vi "Z_info_Save.vi"(7 "Zplane in":i32, 8 "error in (no error)":errorcluster, 11 "AOL_Globals":T1={"Imaging Protocol"=enum."AOL Z-Stack", "Number of POI"=0, "Number of Miniscans"=0, "Number of Trials"=0, "Number of Cycles "=0, "# Averaged Frames"=0, "Laser power (%)"=0, "Pockels"=0.0, "Acquisition Length (sec)"=0.0, "Fill time (us)"=0.0, "POI Dwell time (us)"=0.0, "Miniscan Dwell time per pixel (us)"=0.0, "PMT 1"=0.0, "PMT 2"=0.0, "Back Apperture"=200.0, "Frame Size"=0, "Center Frequency"=0.0, "Field of View"=0.0, "DwellTime (us)"=0.0, "Wavelength (nm)"=0.0, "Zoom"=0.0, "AOL Z"=0.0, "AOL Mode"=enum."Raster", "GridXY"=0.0, "GridZ"=0.0, "TriggerPeriod (sec)"=0.0, "Number of Pixels in Miniscan"=0, "Experiment folder path"=path "", "X centre"=0.0, "Y centre"=0.0, "Angle (degrees)"=0.0, "Plane Mode"=0, "Threshold"=[], "Regenerate Chirps"=FALSE, "Rectangle ROI length (pixels)"=0, "Rectangle ROI height (pixels)"=0, "AOD fill"=0, "Samples Wait after Trigger"=0, "StartUp Delay"=0, "Slip Cycle"=163840, "Add Cycle"=FALSE} {"Plane Mode" items=["XY Plane"]; "Frame Size" items=["100X100"=100, "128X128"=128, "200X200"=200, "256X256"=256, "512X512"=512, "1024x1024"=1024, "2048x2048"=2048]; "Back Apperture" format="%#.6g"; "Pockels" format="%#.6g"; "PMT 2" format="%#.6g"; "PMT 1" format="%#.6g"; "Angle (degrees)" format="%#.6g"; "POI Dwell time (us)" format="%#.6g"}) -> (0 "error out":errorcluster)   [LabVIEW 2013]
uses:
  Typedefs/Controls/AOL_Globals.ctl
  Typedefs/Imaging Protocols enum.ctl
  Typedefs/Frame Size.ctl
  Typedefs/AOL modes.ctl
  Typedefs/Plane Mode.ctl
  <userlib>/My Palettes.lib/Files & paths/Spreadsheet/Write To Spreadsheet File (DBL)-Mod.vi
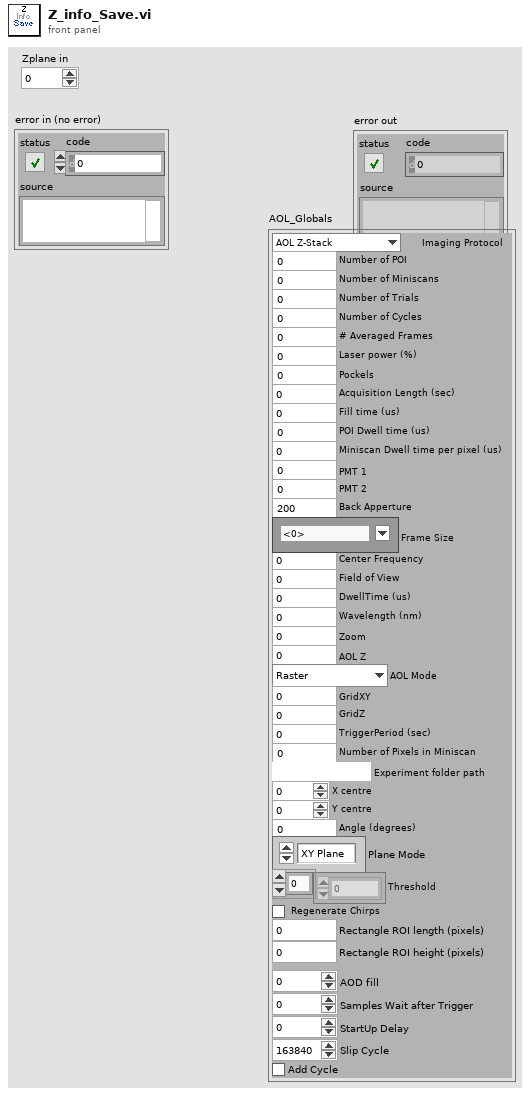
[diagram p1: front panel]
types:
  T1 = typedef "AOL_Globals.ctl" = cluster{"Imaging Protocol":T2, "Number of POI":u16, "Number of Miniscans":u16, "Number of Trials":u16, "Number of Cycles ":u64, "# Averaged Frames":u16, "Laser power (%)":u8, "Pockels":dbl, "Acquisition Length (sec)":dbl, "Fill time (us)":dbl, "POI Dwell time (us)":dbl, "Miniscan Dwell time per pixel (us)":dbl, "PMT 1":dbl, "PMT 2":dbl, "Back Apperture":dbl, "Frame Size":T3, "Center Frequency":dbl, "Field of View":dbl, "DwellTime (us)":dbl, "Wavelength (nm)":dbl, "Zoom":dbl, "AOL Z":dbl, "AOL Mode":T4, "GridXY":dbl, "GridZ":dbl, "TriggerPeriod (sec)":dbl, "Number of Pixels in Miniscan":u16, "Experiment folder path":path, "X centre":dbl, "Y centre":dbl, "Angle (degrees)":dbl, "Plane Mode":T5, "Threshold":u16[], "Regenerate Chirps":bool, "Rectangle ROI length (pixels)":u16, "Rectangle ROI height (pixels)":u16, "AOD fill":u16, "Samples Wait after Trigger":u16, "StartUp Delay":i32, "Slip Cycle":u32, "Add Cycle":bool}
  T2 = typedef "Imaging Protocols enum.ctl" = enum16{"AOL Z-Stack", "Motor Z Stack", "Functional Acquisition", "Single Plane Acquisition", "Volume Acquisition", "Live Imaging", "Live Plane Imaging", "Live Volume Imaging"}
  T3 = typedef "Frame Size.ctl" = u16
  T4 = typedef "AOL modes.ctl" = enum16{"Raster", "Structural", "Pointing", "Mini Scan", "Alignment"}
  T5 = typedef "Plane Mode.ctl" = u16
  T6 = typedef "Fixed strings.ctl" = cluster{"ROI file name":string, "Normalised ROI file name":string, "Zplane Pockels values file name":string, "Functional data folder name":string, "Experiment Header file name":string, "Z-stack images folder name":string, "Groups setup rel. path":string, "Groups text file rel. path":string, "TDMS files folder name (F.img)":string, "TDMS files folder name (V.acq)":string, "TDMS files folder name (Pl.acq)":string, "Cycle rel times sequence file":string, "Dynamically called VIs folder name":string, "Time Series folder base name":string}
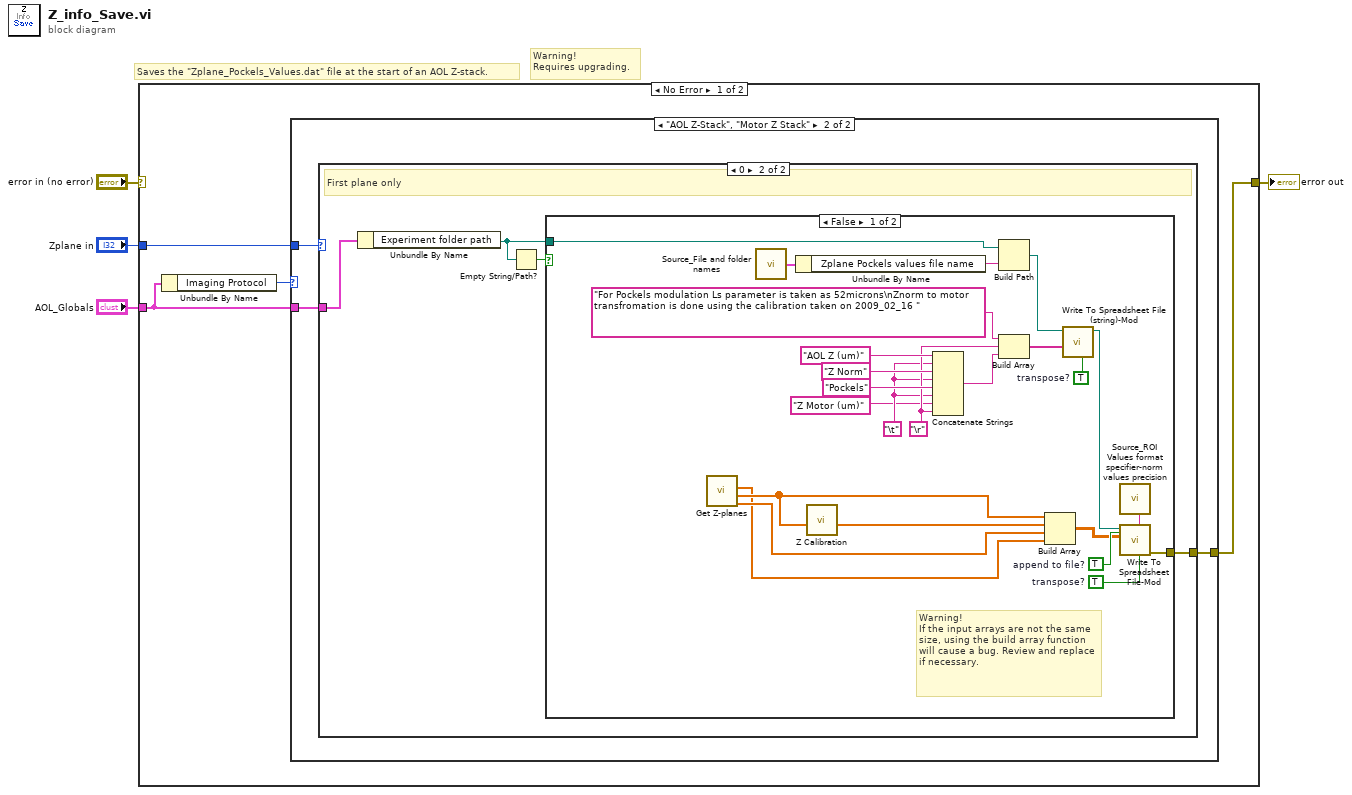
[diagram p0: block diagram]
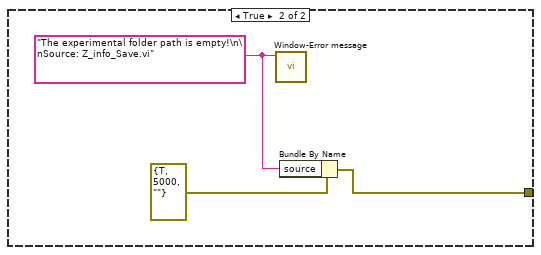
[diagram p4: hidden frame]
diagram:
  # "Warning!\nRequires upgrading."
  # "Saves the \"Zplane_Pockels_Values.dat\" file at the start of an AOL Z-stack."
  n1 = case shown="No Error" "error in (no error)" {
    selector: "error in (no error)" -> [_ w43]
    tunnel: [w5 w43] -> w3
    tunnel: "Zplane in" -> [w7 _]
    tunnel: "AOL_Globals" -> [w6 _]
    frame No Error {
      n2 = Unbundle By Name(w6) -> ("Imaging Protocol"=w8:T2)
      n3 = case shown="\"AOL Z-Stack\", \"Motor Z Stack\"" w8 {
        tunnel: w7 -> [_ w11]
        tunnel: w6 -> [_ w10]
        tunnel: [_ w9] -> w5
        frame Default {
          # "Any protocol other than AOL and Motor Z-stack."
        }
        frame "AOL Z-Stack", "Motor Z Stack" {
          n4 = case shown="0" w11 {
            tunnel: w10 -> [_ w15]
            tunnel: [_ w12] -> w9
            frame Default {
              # "Any plane other than the first one."
            }
            frame 0 {
              # "First plane only"
              n5 = Unbundle By Name(w15) -> ("Experiment folder path"=w14:path)
              n6 = Empty String/Path?(string/path=w14) -> (empty?=w13:bool)
              n7 = case shown="False" w13 {
                tunnel: w14 -> [w37 _]
                tunnel: [w16 w41] -> w12
                frame False {
                  w39 = TRUE  # transpose?
                  w38 = TRUE  # transpose?
                  w33 = TRUE  # append to file?
                  w21 = "\r" ("string")
                  w20 = "\t" ("string")
                  # "Warning!\nIf the input arrays are not the same size, using the build array function will cause a bug. Review and replace if necessary."
                  n8 = call "Get Z-planes.vi"() -> ("Pockels vs. Z (Laser power %)"=w22:dbl[], "Z Planes(um)"=w23:dbl[], "Motor Z Planes(um)"=w17:dbl[])  [unwired: 7 in, 2 out]
                  n9 = call "Source_File and folder names.vi"() -> ("Fixed strings"=w34:T6)  [unwired: 1 in]
                  n10 = Unbundle By Name(w34) -> ("Zplane Pockels values file name"=w35:string)
                  n11 = call "Z Calibration.vi"("Z Planes"=w23) -> ("Norm Z"=w18:dbl[])  [unwired: 7 in, 3 out]
                  n12 = Concatenate Strings("AOL Z (um)" ("string"), w20, "Z Norm" ("string"), w20, "Pockels" ("string"), w20, "Z Motor (um)" ("string"), w21) -> (w27:string)
                  n13 = Build Path(base path=w37, name or relative path=w35) -> (appended path=w32:path)
                  n14 = Build Array("For Pockels modulation Ls parameter is taken as 52microns\nZnorm to motor transfromation is done using the calibration taken on 2009_02_16 " ("element"), w21, w27) -> (w28:string[])
                  n15 = Build Array(w23, w18, w22, w17) -> (w31:dbl[][])
                  n16 = call <userlib>:"Write To Spreadsheet File (string)-Mod.vi"("transpose? (no:F)"=w38, "1D data"=w28, "file path (dialog if empty)"=w32) -> ("new file path (Not A Path if cancelled)"=w30:path)  [unwired: 7 in, 1 out]
                  n17 = call "Source_ROI Values format specifier-norm values precision.vi"() -> ("format (%.3f)"=w36:string)  [unwired: 11 in]
                  n18 = call-poly <userlib>:"Write To Spreadsheet File-Mod.vi"("transpose? (no:F)"=w39, "format (%.3f)"=w36, "append to file? (new file:F)"=w33, "2D data"=w31, "file path (dialog if empty)"=w30) -> ("error out"=w16:errorcluster)  [unwired: 5 in, 1 out]
                }
                frame True {
                  w40 = "The experimental folder path is empty!\n\nSource: Z_info_Save.vi"
                  n19 = call "Window-Error message.vi"("Message"=w40) -> ()  [unwired: 10 in, 1 out]
                  n20 = Bundle By Name(cluster=errorcluster {"status"=TRUE, "code"=5000, "source"=""} ("error out"), "source"=w40) -> (w41:errorcluster)
                }
              }
            }
          }
        }
      }
    }
    frame Error {
    }
  }
  "error out" <- w3
